vi "Publish Model Data.vi"(8 "error in (no error)":errorcluster, 9 "Data to Publish":variant, 10 "Datum Name":string, 11 "IModel in":refnum<class "IModel.lvclass">) -> (0 "error out":errorcluster, 3 "IModel out":refnum<class "IModel.lvclass">)   [LabVIEW 2015, in "IModel.lvlib" / "IModel.lvclass"]
doc: "Publish a datum (value) to the mediator bus. Published data are observable by any actor with access to the mediated bus."
uses:
  IModel.lvclass
  IModel.lvclass/IModel.ctl
  AbstractMessages/PreAddressedMsg/PreAddressedMsg.lvclass/PreAddressedMsg.ctl
  IMediator/IMediator Messages/Publish Msg/Publish Msg.lvclass/Publish Msg.ctl
  <vilib>/ActorFramework/Message Enqueuer/Message Enqueuer.lvclass/Message Enqueuer.ctl
  <vilib>/ActorFramework/Message Enqueuer/Enqueue.vi
  AbstractMessages/PreAddressedMsg/Read Return Address.vi
  <vilib>/ActorFramework/Message Priority Queue/Priority Enqueue.vi
  IMediator/IMediator Messages/Publish Msg/Publish Msg.lvclass
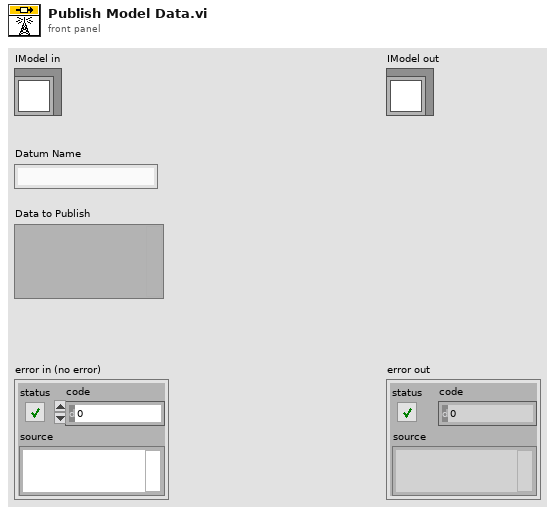
[diagram p1: front panel]
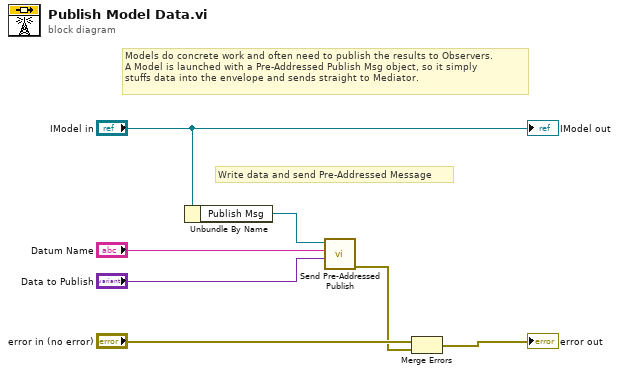
[diagram p0: block diagram]
diagram:
  # "Models do concrete work and often need to publish the results to Observers.\nA Model is launched with a Pre-Addressed Publish Msg object, so it simply\nstuffs data into the envelope and sends straight to Mediator."
  # "Write data and send Pre-Addressed Message"
  n1 = Unbundle By Name("IModel in") -> ("Publish Msg"=w7:refnum<class "Publish Msg.lvclass">)
  n2 = call "Send Pre-Addressed Publish.vi"("Data to Publish"="Data to Publish", "Datum Name"="Datum Name", "Publish Message"=w7) -> ("error out"=w2:errorcluster)  [unwired: 8 in]
  n3 = Merge Errors("error in (no error)", w2) -> (→"error out":errorcluster)
  "IModel out" <- "IModel in"
